vi "Matrix_interpolation.vi"(5 "Constant V for matrixmat":dbl, 6 "Configuration":T1={"Accelerometer Bias"={"X (m/s)"=0.0, "Y (m/s)"=0.0, "Z (m/s)"=0.0}, "Gyroscope Bias"={"X (m/s)"=0.0, "Y (m/s)"=0.0, "Z (m/s)"=0.0}, "Steering Motor Gear Ratio"=611.0, "Steering Pully Gear Ratio"=1.0, "Steering Encoder CPR"=500.0, "Steering Motor Max RPM"=4000.0, "Wheelbase (m)"=1.12, "Fork Angle (rad)"=1.3, "Balancing Controller"={"Kp (/s)"=1.0, "Kd (1)"=1.0}, "Max Allowed Steering Angle (rad)"=0.7, "Task Periods"={"Emergency Stop (us)"=10000, "IMU (us)"=10000, "Steering Motor Encoder (us)"=10000, "State Estimator (us)"=10000, "Balancing Controller (us)"=10000, "GNSS (us)"=10000, "Logging (us)"=50000, "Drive Motor (us)"=100000, "Visualization (us)"=50000}, "Drive Motor Gear Ratio"=0.7, "lr"=0.0, "lf"=0.0, "lambda"=0.0, "k1"=0.0, "k2"=0.0, "e1_max"=0.0, "Ad_tmin"=0.0, "Bd_tmin"=0.0, "C_tmin"=0.0, "D_tmin"=0.0, "Wheel radius"=0.311, "Ad_tmax"=0.95971, "Bd_tmax"=0.01, "C_tmax"=2.20588, "D_tmax"=0.0, "Vmin"=2.20588, "Vmax"=0.0}, 7 "Interpolation activator":bool, 9 "Max":dbl[][](array[numeric]), 10 "Min":dbl[][](array[numeric]), 11 "Vest":dbl) -> (3 "Interpolation output":dbl[][](array[numeric]))   [LabVIEW 2021]
uses:
  Configuration/Configuration.ctl
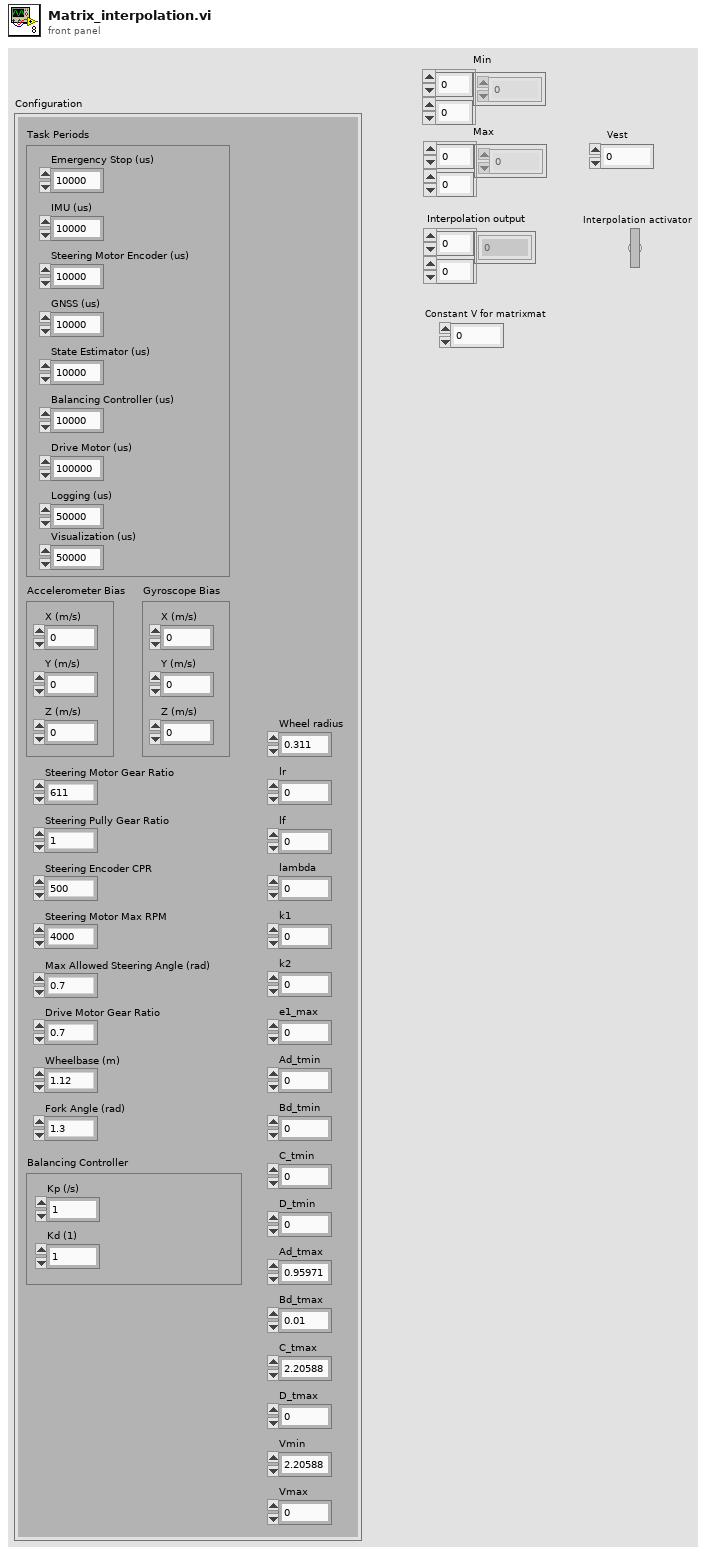
[diagram p1: front panel]
types:
  T1 = typedef "Configuration.ctl" = cluster{"Accelerometer Bias":cluster{"X (m/s)":dbl, "Y (m/s)":dbl, "Z (m/s)":dbl}, "Gyroscope Bias":cluster{"X (m/s)":dbl, "Y (m/s)":dbl, "Z (m/s)":dbl}, "Steering Motor Gear Ratio":dbl, "Steering Pully Gear Ratio":dbl, "Steering Encoder CPR":dbl, "Steering Motor Max RPM":dbl, "Wheelbase (m)":dbl, "Fork Angle (rad)":dbl, "Balancing Controller":cluster{"Kp (/s)":dbl, "Kd (1)":dbl}, "Max Allowed Steering Angle (rad)":dbl, "Task Periods":cluster{"Emergency Stop (us)":i64, "IMU (us)":i64, "Steering Motor Encoder (us)":i64, "State Estimator (us)":i64, "Balancing Controller (us)":i64, "GNSS (us)":i64, "Logging (us)":i64, "Drive Motor (us)":i64, "Visualization (us)":i64}, "Drive Motor Gear Ratio":dbl, "lr":dbl, "lf":dbl, "lambda":dbl, "k1":dbl, "k2":dbl, "e1_max":dbl, "Ad_tmin":dbl, "Bd_tmin":dbl, "C_tmin":dbl, "D_tmin":dbl, "Wheel radius":dbl, "Ad_tmax":dbl, "Bd_tmax":dbl, "C_tmax":dbl, "D_tmax":dbl, "Vmin":dbl, "Vmax":dbl}
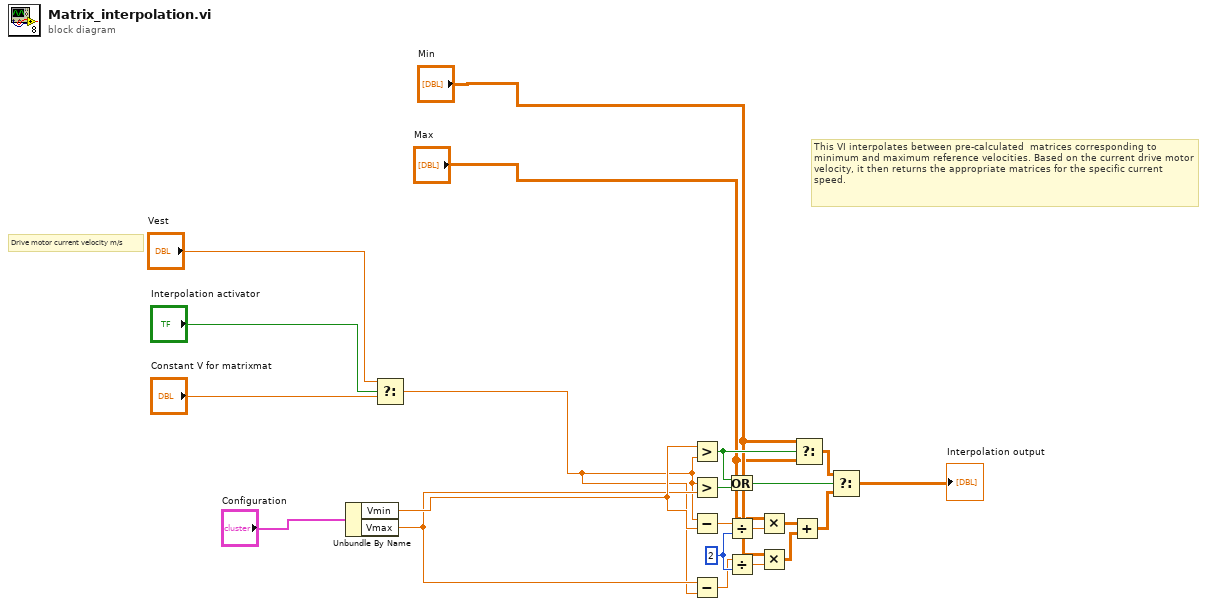
[diagram p0: block diagram]
diagram:
  w13 = 2
  # "This VI interpolates between pre-calculated  matrices corresponding to minimum and maximum reference velocities. Based on the current drive motor velocity, it then returns the appropriate matrices for the specific current speed."
  # "Drive motor current velocity m/s"
  n1 = Unbundle By Name("Configuration") -> ("Vmin"=w6:dbl, "Vmax"=w5:dbl)
  n2 = Select(t="Vest", s="Interpolation activator", f="Constant V for matrixmat") -> (s? t:f=w1:dbl)
  n3 = Greater?(x=w6, y=w1) -> (0:w21:bool)
  n4 = Greater?(x=w1, y=w5) -> (0:w10:bool)
  n5 = Subtract(x=w1, y=w6) -> (x-y=w11:dbl)
  n6 = Subtract(x=w5, y=w1) -> (x-y=w12:dbl)
  n7 = Or(x=w21, y=w10) -> (x .or. y?=w18:bool)
  n8 = Divide(x=w11, y=w13) -> (x/y=w14:dbl)
  n9 = Divide(x=w12, y=w13) -> (x/y=w15:dbl)
  n10 = Multiply(x="Max", y=w14) -> (x*y=w16:dbl[][])
  n11 = Multiply(x="Min", y=w15) -> (x*y=w17:dbl[][])
  n12 = Add(x=w16, y=w17) -> (x+y=w19:dbl[][])
  n13 = Select(t="Min", s=w21, f="Max") -> (s? t:f=w20:dbl[][])
  n14 = Select(t=w20, s=w18, f=w19) -> (s? t:f=→"Interpolation output":dbl[][])
